vi "FTW-Actor-Destroy.vi"(0 "FTW Actor Instance":refnum<class "FTW-ScripterStep-Base.lvclass">, 5 "Force Destroy?":bool=TRUE, 11 "error in":errorcluster) -> (15 "error out":errorcluster)   [LabVIEW 2015]
uses:
  source/actor/Connector/FTW-ActorConnector.lvclass
  FTW-ScripterStep-Base.lvclass
panel:
  # "Inputs"
  # "Outputs"
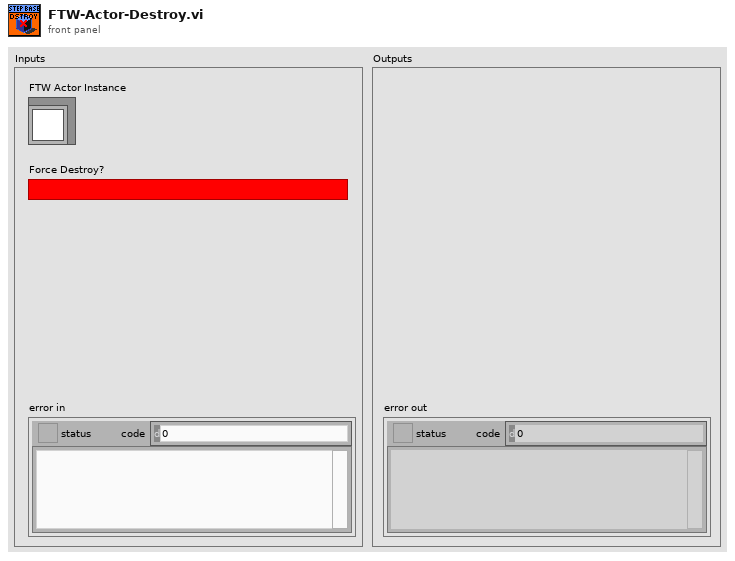
[diagram p1: front panel]
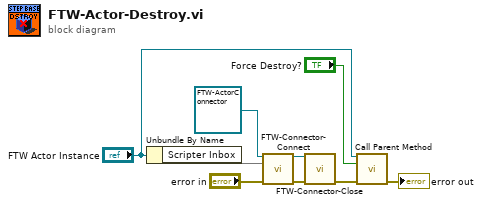
[diagram p0: block diagram]
diagram:
  n1 = Unbundle By Name("FTW Actor Instance") -> ("Scripter Inbox"=w4)
  n2 = call-dynamic "FTW-Connector-Connect.vi"("FTW Actor Connector Type"=refnum<class "FTW-ActorConnector.lvclass"> refnum, "Instance Inbox Address"=w4, "error in"="error in") -> ("FTW Actor Connector"=w1:refnum<class "FTW-ActorConnector.lvclass">, "error out"=w5:errorcluster)  [unwired: 11 in]
  n3 = call-dynamic "FTW-Connector-Close.vi"("FTW Actor Connector"=w1, "error in"=w5) -> ("error out"=w2:errorcluster)  [unwired: 13 in]
  n4 = call-parent "Call Parent Method"("FTW Actor Instance"="FTW Actor Instance", "Force Destroy?"="Force Destroy?", "error in"=w2) -> ("error out"=→"error out":errorcluster)  [unwired: 12 in]
